vi "BCU参数读取-Auto.vi"(8 "CAN端口":u16(ring), 9 "设备索引号":u16(ring), 10 "CAN卡类型":u32(ring)=21, 11 "Myindex":dbl=1.0) -> (3 "成功":bool)   [LabVIEW 2013] (continued)
                        n3743 = Boolean To (0,1)(Boolean=w5434) -> (0, 1=w5432:i16)
                        n3744 = Quotient & Remainder(x=w5429, y=w5430) -> (x-y*floor(x/y)=w5426:dbl)  [unwired: 1 out]
                        n3745 = Build Array(i16 170 ("元素"), w5432, w5426, w5425, w5424, w5423, 0.0 ("元素")) -> (w5435:dbl[])
                        n3746 = call "多帧发送机制(EV05).vi"("can卡类型"=w5439, "设备索引号"=w5438, "CAN端口"=w5437, "命令"=w5420, "板号"=u8 0, "命令序号"=w5421, "输入数据"=w5435) -> ()  [unwired: 2 in, 11 out]
                        n3747 = local write "命令序号"(w5421) -> ()
                        n3748 = local write "命令"(w5420) -> ()
                      }
                    }
                    n3749 = local write "控制1"(TRUE ("控制1")) -> ()
                    n3750 = local write "写?"(FALSE ("写?")) -> ()
                    n3751 = local write "消除"(TRUE ("消除")) -> ()
                    n3752 = global write "EV05全局变量1.vi" "流控帧 2"(TRUE ("流控帧 2")) -> ()
                    n3753 = global write "EV05全局变量1.vi" "流控帧"(FALSE ("流控帧")) -> ()
                  }
                  frame #2 {
                    n3754 = flat-sequence {
                      tunnel: [w5441] -> w5440
                      tunnel: w5440 -> [w5448]
                      frame #0 {
                        n3755 = while {
                          tunnel: [w5442] -> w5441
                          i -> [w5446]
                          stop <- w5443 stop-if-true
                          n3756 = local read "继电器超时处理"() -> (w5442:bool)
                          n3757 = Greater Or Equal?(x=w5446, y=20) -> (x >= y?=w5444:bool)
                          n3758 = Wait Until Next ms Multiple(millisecond multiple=u32 100 ("毫秒倍数")) -> ()  [unwired: 1 out]
                          n3759 = Or(x=w5442, y=w5444) -> (x .or. y?=w5443:bool)
                        }
                      }
                      frame #1 {
                        n3760 = case shown="真" w5448 {
                          frame False {
                            n3761 = One Button Dialog(message="继电器处理超时" ("消息"), button name ("OK")="是" ("按钮名称（“确定”）")) -> ()  [unwired: 1 out]
                          }
                          frame True {
                            w5451 = TRUE ("清BUFF")
                            n3762 = local write "正级继电器"(w5451) -> ()
                            n3763 = local write "负级继电器"(w5451) -> ()
                            n3764 = local write "充电继电器"(w5451) -> ()
                            n3765 = local write "加热继电器"(w5451) -> ()
                            n3766 = local write "风机继电器"(w5451) -> ()
                            n3767 = local write "预充电继电器"(w5451) -> ()
                          }
                        }
                      }
                    }
                  }
                }
              }
            }
          }
          event "继电器全关": Value Change {
            n3768 = event-data() -> ("NewVal"=w5452:bool)  [unwired: 6 out]
            n3769 = case shown="真" w5452 {
              tunnel: w5452 -> [_ w5455]
              frame False {
              }
              frame True {
                n3770 = stacked-sequence {
                  tunnel: w5455 -> [_ w5465 _]
                  frame #0 {
                    w5456 = TRUE ("清BUFF")
                    n3771 = local write "正级继电器"(w5456) -> ()
                    n3772 = local write "负级继电器"(w5456) -> ()
                    n3773 = local write "充电继电器"(w5456) -> ()
                    n3774 = local write "加热继电器"(w5456) -> ()
                    n3775 = local write "风机继电器"(w5456) -> ()
                    n3776 = local write "预充电继电器"(w5456) -> ()
                    n3777 = local write "继电器超时处理"(FALSE ("继电器超时处理")) -> ()
                    n3778 = local write "主从选择"(enum32{"主板", "从板"}."主板" ("主从选择")) -> ()
                    n3779 = global write "EV05全局变量1.vi" "流控帧"(FALSE ("流控帧")) -> ()
                    n3780 = local write "清BUFF"(FALSE ("清BUFF")) -> ()
                  }
                  frame #1 {
                    n3781 = case shown="真" w5465 {
                      selector: w5465 -> [_ w5480]
                      frame False {
                      }
                      frame True {
                        w5476 = 256.0 ("y")
                        w5467 = u32 1 ("命令序号")
                        w5466 = u8 192 ("命令")
                        n3782 = local read "动作保持时间"() -> (w5477:dbl)
                        n3783 = Quotient & Remainder(x=w5477, y=w5476) -> (x-y*floor(x/y)=w5469:dbl, floor(x/y)=w5473:dbl)
                        n3784 = Quotient & Remainder(x=w5473, y=w5476) -> (x-y*floor(x/y)=w5470:dbl, floor(x/y)=w5474:dbl)
                        n3785 = Quotient & Remainder(x=w5474, y=w5476) -> (x-y*floor(x/y)=w5471:dbl, floor(x/y)=w5475:dbl)
                        n3786 = local read "设备索引号"() -> (w5484:u16)
                        n3787 = local read "CAN卡类型"() -> (w5485:u32)
                        n3788 = local read "CAN端口"() -> (w5483:u16)
                        n3789 = Boolean To (0,1)(Boolean=w5480) -> (0, 1=w5478:i16)
                        n3790 = Quotient & Remainder(x=w5475, y=w5476) -> (x-y*floor(x/y)=w5472:dbl)  [unwired: 1 out]
                        n3791 = Build Array(i16 85 ("元素"), w5478, w5472, w5471, w5470, w5469, 0.0 ("元素")) -> (w5481:dbl[])
                        n3792 = call "多帧发送机制(EV05).vi"("can卡类型"=w5485, "设备索引号"=w5484, "CAN端口"=w5483, "命令"=w5466, "板号"=u8 0, "命令序号"=w5467, "输入数据"=w5481) -> ()  [unwired: 2 in, 11 out]
                        n3793 = local write "命令序号"(w5467) -> ()
                        n3794 = local write "命令"(w5466) -> ()
                      }
                    }
                    n3795 = local write "控制1"(TRUE ("控制1")) -> ()
                    n3796 = local write "写?"(FALSE ("写?")) -> ()
                    n3797 = local write "消除"(TRUE ("消除")) -> ()
                    n3798 = global write "EV05全局变量1.vi" "流控帧 2"(TRUE ("流控帧 2")) -> ()
                  }
                  frame #2 {
                    n3799 = flat-sequence {
                      tunnel: [w5487] -> w5486
                      tunnel: w5486 -> [w5494]
                      frame #0 {
                        n3800 = while {
                          tunnel: [w5488] -> w5487
                          i -> [w5492]
                          stop <- w5489 stop-if-true
                          n3801 = local read "继电器超时处理"() -> (w5488:bool)
                          n3802 = Greater Or Equal?(x=w5492, y=20) -> (x >= y?=w5490:bool)
                          n3803 = Wait Until Next ms Multiple(millisecond multiple=u32 100 ("毫秒倍数")) -> ()  [unwired: 1 out]
                          n3804 = Or(x=w5488, y=w5490) -> (x .or. y?=w5489:bool)
                        }
                      }
                      frame #1 {
                        n3805 = case shown="真" w5494 {
                          frame False {
                            n3806 = One Button Dialog(message="继电器处理超时" ("消息"), button name ("OK")="是" ("按钮名称（“确定”）")) -> ()  [unwired: 1 out]
                          }
                          frame True {
                            w5497 = FALSE ("清BUFF")
                            n3807 = local write "正级继电器"(w5497) -> ()
                            n3808 = local write "负级继电器"(w5497) -> ()
                            n3809 = local write "充电继电器"(w5497) -> ()
                            n3810 = local write "加热继电器"(w5497) -> ()
                            n3811 = local write "风机继电器"(w5497) -> ()
                            n3812 = local write "预充电继电器"(w5497) -> ()
                          }
                        }
                      }
                    }
                  }
                }
              }
            }
          }
          event "控制按键全为开": Value Change {
            n3813 = event-data() -> ("NewVal"=w5498:bool)  [unwired: 6 out]
            n3814 = case shown="真" w5498 {
              frame False {
              }
              frame True {
                w5499 = TRUE ("正级继电器")
                n3815 = local write "加热继电器(从)"(w5499) -> ()
                n3816 = local write "风机继电器(从)"(w5499) -> ()
                n3817 = local write "DO1 2"(w5499) -> ()
                n3818 = local write "DO1"(w5499) -> ()
                n3819 = local write "DO2"(w5499) -> ()
                n3820 = local write "正级继电器"(w5499) -> ()
                n3821 = local write "负级继电器"(w5499) -> ()
                n3822 = local write "加热继电器"(w5499) -> ()
                n3823 = local write "预充电继电器"(w5499) -> ()
                n3824 = local write "充电继电器"(w5499) -> ()
                n3825 = local write "风机继电器"(w5499) -> ()
              }
            }
          }
          event "控制按键全为关": Value Change {
            n3826 = event-data() -> ("NewVal"=w5500:bool)  [unwired: 6 out]
            n3827 = case shown="真" w5500 {
              frame False {
              }
              frame True {
                w5501 = FALSE ("正级继电器")
                n3828 = local write "加热继电器(从)"(w5501) -> ()
                n3829 = local write "风机继电器(从)"(w5501) -> ()
                n3830 = local write "DO1 2"(w5501) -> ()
                n3831 = local write "DO1"(w5501) -> ()
                n3832 = local write "DO2"(w5501) -> ()
                n3833 = local write "正级继电器"(w5501) -> ()
                n3834 = local write "负级继电器"(w5501) -> ()
                n3835 = local write "加热继电器"(w5501) -> ()
                n3836 = local write "预充电继电器"(w5501) -> ()
                n3837 = local write "充电继电器"(w5501) -> ()
                n3838 = local write "风机继电器"(w5501) -> ()
              }
            }
          }
          event "正级继电器": Value Change {
            n3839 = event-data() -> ("NewVal"=w5502:bool)  [unwired: 6 out]
            n3840 = stacked-sequence {
              tunnel: w5502 -> [_ w5515 _]
              frame #0 {
                w5505 = FALSE ("清BUFF")
                n3841 = local write "继电器超时处理"(FALSE ("继电器超时处理")) -> ()
                n3842 = local write "主从选择"(enum32{"主板", "从板"}."主板" ("主从选择")) -> ()
                n3843 = local write "正级继电器 12"(w5505) -> ()
                n3844 = local write "清BUFF"(w5505) -> ()
              }
              frame #1 {
                n3845 = case shown="假" w5515 {
                  selector: w5515 -> [w5530 w5550]
                  tunnel: [w5529 w5549] -> w5514
                  tunnel: [w5517 w5537] -> w5509
                  frame False {
                    w5525 = 256.0 ("y")
                    w5517 = u32 1 ("命令序号")
                    w5529 = u8 192 ("命令")
                    n3846 = local read "动作保持时间"() -> (w5526:dbl)
                    n3847 = Quotient & Remainder(x=w5526, y=w5525) -> (x-y*floor(x/y)=w5518:dbl, floor(x/y)=w5522:dbl)
                    n3848 = Quotient & Remainder(x=w5522, y=w5525) -> (x-y*floor(x/y)=w5519:dbl, floor(x/y)=w5523:dbl)
                    n3849 = Quotient & Remainder(x=w5523, y=w5525) -> (x-y*floor(x/y)=w5520:dbl, floor(x/y)=w5524:dbl)
                    n3850 = local read "设备索引号"() -> (w5534:u16)
                    n3851 = local read "CAN卡类型"() -> (w5535:u32)
                    n3852 = local read "CAN端口"() -> (w5533:u16)
                    n3853 = Boolean To (0,1)(Boolean=w5530) -> (0, 1=w5527:i16)
                    n3854 = Quotient & Remainder(x=w5524, y=w5525) -> (x-y*floor(x/y)=w5521:dbl)  [unwired: 1 out]
                    n3855 = Build Array(i16 1 ("元素"), w5527, w5521, w5520, w5519, w5518, 0.0 ("元素")) -> (w5531:dbl[])
                    n3856 = call "多帧发送机制(EV05).vi"("can卡类型"=w5535, "设备索引号"=w5534, "CAN端口"=w5533, "命令"=w5529, "板号"=u8 0, "命令序号"=w5517, "输入数据"=w5531) -> ()  [unwired: 2 in, 11 out]
                  }
                  frame True {
                    w5545 = 256.0 ("y")
                    w5537 = u32 1 ("命令序号")
                    w5549 = u8 192 ("命令")
                    n3857 = local read "动作保持时间"() -> (w5546:dbl)
                    n3858 = Quotient & Remainder(x=w5546, y=w5545) -> (x-y*floor(x/y)=w5538:dbl, floor(x/y)=w5542:dbl)
                    n3859 = Quotient & Remainder(x=w5542, y=w5545) -> (x-y*floor(x/y)=w5539:dbl, floor(x/y)=w5543:dbl)
                    n3860 = Quotient & Remainder(x=w5543, y=w5545) -> (x-y*floor(x/y)=w5540:dbl, floor(x/y)=w5544:dbl)
                    n3861 = local read "设备索引号"() -> (w5554:u16)
                    n3862 = local read "CAN卡类型"() -> (w5555:u32)
                    n3863 = local read "CAN端口"() -> (w5553:u16)
                    n3864 = Boolean To (0,1)(Boolean=w5550) -> (0, 1=w5547:i16)
                    n3865 = Quotient & Remainder(x=w5544, y=w5545) -> (x-y*floor(x/y)=w5541:dbl)  [unwired: 1 out]
                    n3866 = Build Array(i16 1 ("元素"), w5547, w5541, w5540, w5539, w5538, 0.0 ("元素")) -> (w5551:dbl[])
                    n3867 = call "多帧发送机制(EV05).vi"("can卡类型"=w5555, "设备索引号"=w5554, "CAN端口"=w5553, "命令"=w5549, "板号"=u8 0, "命令序号"=w5537, "输入数据"=w5551) -> ()  [unwired: 2 in, 11 out]
                  }
                }
                n3868 = local write "命令序号"(w5509) -> ()
                n3869 = local write "命令"(w5514) -> ()
                n3870 = local write "控制1"(TRUE ("控制1")) -> ()
                n3871 = local write "写?"(FALSE ("写?")) -> ()
                n3872 = global write "EV05全局变量1.vi" "流控帧"(FALSE ("流控帧")) -> ()
                n3873 = local write "消除"(TRUE ("消除")) -> ()
                n3874 = global write "EV05全局变量1.vi" "流控帧 2"(TRUE ("流控帧 2")) -> ()
              }
              frame #2 {
                n3875 = flat-sequence {
                  tunnel: [w5557] -> w5556
                  tunnel: w5556 -> [w5564]
                  frame #0 {
                    n3876 = while {
                      tunnel: [w5558] -> w5557
                      i -> [w5562]
                      stop <- w5559 stop-if-true
                      n3877 = local read "继电器超时处理"() -> (w5558:bool)
                      n3878 = Greater Or Equal?(x=w5562, y=20) -> (x >= y?=w5560:bool)
                      n3879 = Wait Until Next ms Multiple(millisecond multiple=u32 100 ("毫秒倍数")) -> ()  [unwired: 1 out]
                      n3880 = Or(x=w5558, y=w5560) -> (x .or. y?=w5559:bool)
                    }
                  }
                  frame #1 {
                    n3881 = case shown="假" w5564 {
                      frame False {
                        n3882 = local read "正级继电器"() -> (w5566:bool)
                        n3883 = Not(x=w5566) -> (.not. x?=w5565:bool)
                        n3884 = local write "正级继电器"(w5565) -> ()
                        n3885 = One Button Dialog(message="继电器处理超时" ("消息"), button name ("OK")="是" ("按钮名称（“确定”）")) -> ()  [unwired: 1 out]
                      }
                      frame True {
                      }
                    }
                  }
                }
              }
            }
          }
          event "负级继电器": Value Change {
            n3886 = event-data() -> ("NewVal"=w5569:bool)  [unwired: 6 out]
            n3887 = stacked-sequence {
              tunnel: w5569 -> [_ w5582 _]
              frame #0 {
                w5572 = FALSE ("继电器超时处理")
                n3888 = local write "继电器超时处理"(w5572) -> ()
                n3889 = local write "正级继电器 2"(w5572) -> ()
                n3890 = local write "主从选择"(enum32{"主板", "从板"}."主板" ("主从选择")) -> ()
              }
              frame #1 {
                n3891 = case shown="假" w5582 {
                  selector: w5582 -> [w5596 w5616]
                  tunnel: [w5595 w5615] -> w5581
                  tunnel: [w5584 w5604] -> w5576
                  frame False {
                    w5592 = 256.0 ("y")
                    w5584 = u32 1 ("命令序号")
                    w5595 = u8 192 ("命令")
                    n3892 = local read "动作保持时间"() -> (w5593:dbl)
                    n3893 = Quotient & Remainder(x=w5593, y=w5592) -> (x-y*floor(x/y)=w5585:dbl, floor(x/y)=w5589:dbl)
                    n3894 = Quotient & Remainder(x=w5589, y=w5592) -> (x-y*floor(x/y)=w5586:dbl, floor(x/y)=w5590:dbl)
                    n3895 = Quotient & Remainder(x=w5590, y=w5592) -> (x-y*floor(x/y)=w5587:dbl, floor(x/y)=w5591:dbl)
                    n3896 = Quotient & Remainder(x=w5591, y=w5592) -> (x-y*floor(x/y)=w5588:dbl)  [unwired: 1 out]
                    n3897 = Boolean To (0,1)(Boolean=w5596) -> (0, 1=w5594:i16)
                    n3898 = local read "设备索引号"() -> (w5601:u16)
                    n3899 = local read "CAN卡类型"() -> (w5602:u32)
                    n3900 = local read "CAN端口"() -> (w5600:u16)
                    n3901 = Build Array(i16 2 ("元素"), w5594, w5588, w5587, w5586, w5585, 0.0 ("元素")) -> (w5598:dbl[])
                    n3902 = call "多帧发送机制(EV05).vi"("can卡类型"=w5602, "设备索引号"=w5601, "CAN端口"=w5600, "命令"=w5595, "板号"=u8 0, "命令序号"=w5584, "输入数据"=w5598) -> ()  [unwired: 2 in, 11 out]
                  }
                  frame True {
                    w5612 = 256.0 ("y")
                    w5604 = u32 1 ("命令序号")
                    w5615 = u8 192 ("命令")
                    n3903 = local read "动作保持时间"() -> (w5613:dbl)
                    n3904 = Quotient & Remainder(x=w5613, y=w5612) -> (x-y*floor(x/y)=w5605:dbl, floor(x/y)=w5609:dbl)
                    n3905 = Quotient & Remainder(x=w5609, y=w5612) -> (x-y*floor(x/y)=w5606:dbl, floor(x/y)=w5610:dbl)
                    n3906 = Quotient & Remainder(x=w5610, y=w5612) -> (x-y*floor(x/y)=w5607:dbl, floor(x/y)=w5611:dbl)
                    n3907 = Quotient & Remainder(x=w5611, y=w5612) -> (x-y*floor(x/y)=w5608:dbl)  [unwired: 1 out]
                    n3908 = Boolean To (0,1)(Boolean=w5616) -> (0, 1=w5614:i16)
                    n3909 = local read "设备索引号"() -> (w5621:u16)
                    n3910 = local read "CAN卡类型"() -> (w5622:u32)
                    n3911 = local read "CAN端口"() -> (w5620:u16)
                    n3912 = Build Array(i16 2 ("元素"), w5614, w5608, w5607, w5606, w5605, 0.0 ("元素")) -> (w5618:dbl[])
                    n3913 = call "多帧发送机制(EV05).vi"("can卡类型"=w5622, "设备索引号"=w5621, "CAN端口"=w5620, "命令"=w5615, "板号"=u8 0, "命令序号"=w5604, "输入数据"=w5618) -> ()  [unwired: 2 in, 11 out]
                  }
                }
                n3914 = local write "命令"(w5581) -> ()
                n3915 = local write "命令序号"(w5576) -> ()
                n3916 = local write "清BUFF"(FALSE ("清BUFF")) -> ()
                n3917 = global write "EV05全局变量1.vi" "流控帧"(FALSE ("流控帧")) -> ()
                n3918 = local write "控制1"(TRUE ("控制1")) -> ()
                n3919 = global write "EV05全局变量1.vi" "流控帧 2"(TRUE ("流控帧 2")) -> ()
                n3920 = local write "写?"(FALSE ("写?")) -> ()
                n3921 = local write "消除"(TRUE ("消除")) -> ()
              }
              frame #2 {
                n3922 = flat-sequence {
                  tunnel: [w5624] -> w5623
                  tunnel: w5623 -> [w5631]
                  frame #0 {
                    n3923 = while {
                      tunnel: [w5625] -> w5624
                      i -> [w5629]
                      stop <- w5626 stop-if-true
                      n3924 = local read "继电器超时处理"() -> (w5625:bool)
                      n3925 = Greater Or Equal?(x=w5629, y=20) -> (x >= y?=w5627:bool)
                      n3926 = Wait Until Next ms Multiple(millisecond multiple=u32 100 ("毫秒倍数")) -> ()  [unwired: 1 out]
                      n3927 = Or(x=w5625, y=w5627) -> (x .or. y?=w5626:bool)
                    }
                  }
                  frame #1 {
                    n3928 = case shown="假" w5631 {
                      frame False {
                        n3929 = local read "负级继电器"() -> (w5632:bool)
                        n3930 = Not(x=w5632) -> (.not. x?=w5633:bool)
                        n3931 = local write "负级继电器"(w5633) -> ()
                        n3932 = One Button Dialog(message="继电器处理超时" ("消息"), button name ("OK")="是" ("按钮名称（“确定”）")) -> ()  [unwired: 1 out]
                      }
                      frame True {
                      }
                    }
                  }
                }
              }
            }
          }
          event "预充电继电器": Value Change {
            n3933 = event-data() -> ("NewVal"=w5636:bool)  [unwired: 6 out]
            n3934 = stacked-sequence {
              tunnel: w5636 -> [_ w5649 _]
              frame #0 {
                w5640 = FALSE ("继电器超时处理")
                n3935 = local write "继电器超时处理"(w5640) -> ()
                n3936 = local write "正级继电器 3"(w5640) -> ()
                n3937 = global write "EV05全局变量1.vi" "流控帧"(FALSE ("流控帧")) -> ()
                n3938 = local write "主从选择"(enum32{"主板", "从板"}."主板" ("主从选择")) -> ()
              }
              frame #1 {
                n3939 = case shown="假" w5649 {
                  selector: w5649 -> [w5663 w5683]
                  tunnel: [w5662 w5682] -> w5648
                  tunnel: [w5651 w5671] -> w5643
                  frame False {
                    w5659 = 256.0 ("y")
                    w5651 = u32 1 ("命令序号")
                    w5662 = u8 192 ("命令")
                    n3940 = local read "动作保持时间"() -> (w5660:dbl)
                    n3941 = Quotient & Remainder(x=w5660, y=w5659) -> (x-y*floor(x/y)=w5652:dbl, floor(x/y)=w5656:dbl)
                    n3942 = Quotient & Remainder(x=w5656, y=w5659) -> (x-y*floor(x/y)=w5653:dbl, floor(x/y)=w5657:dbl)
                    n3943 = Quotient & Remainder(x=w5657, y=w5659) -> (x-y*floor(x/y)=w5654:dbl, floor(x/y)=w5658:dbl)
                    n3944 = Quotient & Remainder(x=w5658, y=w5659) -> (x-y*floor(x/y)=w5655:dbl)  [unwired: 1 out]
                    n3945 = Boolean To (0,1)(Boolean=w5663) -> (0, 1=w5661:i16)
                    n3946 = local read "设备索引号"() -> (w5668:u16)
                    n3947 = local read "CAN卡类型"() -> (w5669:u32)
                    n3948 = local read "CAN端口"() -> (w5667:u16)
                    n3949 = Build Array(i16 3 ("元素"), w5661, w5655, w5654, w5653, w5652, 0.0 ("元素")) -> (w5665:dbl[])
                    n3950 = call "多帧发送机制(EV05).vi"("can卡类型"=w5669, "设备索引号"=w5668, "CAN端口"=w5667, "命令"=w5662, "板号"=u8 0, "命令序号"=w5651, "输入数据"=w5665) -> ()  [unwired: 2 in, 11 out]
                  }
                  frame True {
                    w5679 = 256.0 ("y")
                    w5671 = u32 1 ("命令序号")
                    w5682 = u8 192 ("命令")
                    n3951 = local read "动作保持时间"() -> (w5680:dbl)
                    n3952 = Quotient & Remainder(x=w5680, y=w5679) -> (x-y*floor(x/y)=w5672:dbl, floor(x/y)=w5676:dbl)
                    n3953 = Quotient & Remainder(x=w5676, y=w5679) -> (x-y*floor(x/y)=w5673:dbl, floor(x/y)=w5677:dbl)
                    n3954 = Quotient & Remainder(x=w5677, y=w5679) -> (x-y*floor(x/y)=w5674:dbl, floor(x/y)=w5678:dbl)
                    n3955 = Quotient & Remainder(x=w5678, y=w5679) -> (x-y*floor(x/y)=w5675:dbl)  [unwired: 1 out]
                    n3956 = Boolean To (0,1)(Boolean=w5683) -> (0, 1=w5681:i16)
                    n3957 = local read "设备索引号"() -> (w5688:u16)
                    n3958 = local read "CAN卡类型"() -> (w5689:u32)
                    n3959 = local read "CAN端口"() -> (w5687:u16)
                    n3960 = Build Array(i16 3 ("元素"), w5681, w5675, w5674, w5673, w5672, 0.0 ("元素")) -> (w5685:dbl[])
                    n3961 = call "多帧发送机制(EV05).vi"("can卡类型"=w5689, "设备索引号"=w5688, "CAN端口"=w5687, "命令"=w5682, "板号"=u8 0, "命令序号"=w5671, "输入数据"=w5685) -> ()  [unwired: 2 in, 11 out]
                  }
                }
                n3962 = local write "命令序号"(w5643) -> ()
                n3963 = local write "清BUFF"(FALSE ("清BUFF")) -> ()
                n3964 = local write "控制1"(TRUE ("控制1")) -> ()
                n3965 = global write "EV05全局变量1.vi" "流控帧 2"(TRUE ("流控帧 2")) -> ()
                n3966 = local write "消除"(TRUE ("消除")) -> ()
                n3967 = local write "命令"(w5648) -> ()
                n3968 = local write "写?"(FALSE ("写?")) -> ()
              }
              frame #2 {
                n3969 = flat-sequence {
                  tunnel: [w5691] -> w5690
                  tunnel: w5690 -> [w5698]
                  frame #0 {
                    n3970 = while {
                      tunnel: [w5692] -> w5691
                      i -> [w5696]
                      stop <- w5693 stop-if-true
                      n3971 = local read "继电器超时处理"() -> (w5692:bool)
                      n3972 = Greater Or Equal?(x=w5696, y=20) -> (x >= y?=w5694:bool)
                      n3973 = Wait Until Next ms Multiple(millisecond multiple=u32 100 ("毫秒倍数")) -> ()  [unwired: 1 out]
                      n3974 = Or(x=w5692, y=w5694) -> (x .or. y?=w5693:bool)
                    }
                  }
                  frame #1 {
                    n3975 = case shown="假" w5698 {
                      frame False {
                        n3976 = local read "预充电继电器"() -> (w5699:bool)
                        n3977 = Not(x=w5699) -> (.not. x?=w5700:bool)
                        n3978 = local write "预充电继电器"(w5700) -> ()
                        n3979 = One Button Dialog(message="继电器处理超时" ("消息"), button name ("OK")="是" ("按钮名称（“确定”）")) -> ()  [unwired: 1 out]
                      }
                      frame True {
                      }
                    }
                  }
                }
              }
            }
          }
          event "加热继电器": Value Change {
            n3980 = event-data() -> ("NewVal"=w5703:bool)  [unwired: 6 out]
            n3981 = stacked-sequence {
              tunnel: w5703 -> [_ w5716 _]
              frame #0 {
                w5707 = FALSE ("继电器超时处理")
                n3982 = local write "继电器超时处理"(w5707) -> ()
                n3983 = local write "正级继电器 5"(w5707) -> ()
                n3984 = global write "EV05全局变量1.vi" "流控帧"(FALSE ("流控帧")) -> ()
                n3985 = local write "主从选择"(enum32{"主板", "从板"}."主板" ("主从选择")) -> ()
              }
              frame #1 {
                n3986 = case shown="假" w5716 {
                  selector: w5716 -> [w5730 w5750]
                  tunnel: [w5729 w5749] -> w5715
                  tunnel: [w5718 w5738] -> w5710
                  frame False {
                    w5726 = 256.0 ("y")
                    w5718 = u32 1 ("命令序号")
                    w5729 = u8 192 ("命令")
                    n3987 = local read "动作保持时间"() -> (w5727:dbl)
                    n3988 = Quotient & Remainder(x=w5727, y=w5726) -> (x-y*floor(x/y)=w5719:dbl, floor(x/y)=w5723:dbl)
                    n3989 = Quotient & Remainder(x=w5723, y=w5726) -> (x-y*floor(x/y)=w5720:dbl, floor(x/y)=w5724:dbl)
                    n3990 = Quotient & Remainder(x=w5724, y=w5726) -> (x-y*floor(x/y)=w5721:dbl, floor(x/y)=w5725:dbl)
                    n3991 = Quotient & Remainder(x=w5725, y=w5726) -> (x-y*floor(x/y)=w5722:dbl)  [unwired: 1 out]
                    n3992 = Boolean To (0,1)(Boolean=w5730) -> (0, 1=w5728:i16)
                    n3993 = local read "设备索引号"() -> (w5735:u16)
                    n3994 = local read "CAN卡类型"() -> (w5736:u32)
                    n3995 = local read "CAN端口"() -> (w5734:u16)
                    n3996 = Build Array(i16 4 ("元素"), w5728, w5722, w5721, w5720, w5719, 0.0 ("元素")) -> (w5732:dbl[])
                    n3997 = call "多帧发送机制(EV05).vi"("can卡类型"=w5736, "设备索引号"=w5735, "CAN端口"=w5734, "命令"=w5729, "板号"=u8 0, "命令序号"=w5718, "输入数据"=w5732) -> ()  [unwired: 2 in, 11 out]
                  }
                  frame True {
                    w5746 = 256.0 ("y")
                    w5738 = u32 1 ("命令序号")
                    w5749 = u8 192 ("命令")
                    n3998 = local read "动作保持时间"() -> (w5747:dbl)
                    n3999 = Quotient & Remainder(x=w5747, y=w5746) -> (x-y*floor(x/y)=w5739:dbl, floor(x/y)=w5743:dbl)
                    n4000 = Quotient & Remainder(x=w5743, y=w5746) -> (x-y*floor(x/y)=w5740:dbl, floor(x/y)=w5744:dbl)
                    n4001 = Quotient & Remainder(x=w5744, y=w5746) -> (x-y*floor(x/y)=w5741:dbl, floor(x/y)=w5745:dbl)
                    n4002 = Quotient & Remainder(x=w5745, y=w5746) -> (x-y*floor(x/y)=w5742:dbl)  [unwired: 1 out]
                    n4003 = Boolean To (0,1)(Boolean=w5750) -> (0, 1=w5748:i16)
                    n4004 = local read "设备索引号"() -> (w5755:u16)
                    n4005 = local read "CAN卡类型"() -> (w5756:u32)
                    n4006 = local read "CAN端口"() -> (w5754:u16)
                    n4007 = Build Array(i16 4 ("元素"), w5748, w5742, w5741, w5740, w5739, 0.0 ("元素")) -> (w5752:dbl[])
                    n4008 = call "多帧发送机制(EV05).vi"("can卡类型"=w5756, "设备索引号"=w5755, "CAN端口"=w5754, "命令"=w5749, "板号"=u8 0, "命令序号"=w5738, "输入数据"=w5752) -> ()  [unwired: 2 in, 11 out]
                  }
                }
                n4009 = local write "命令序号"(w5710) -> ()
                n4010 = local write "清BUFF"(FALSE ("清BUFF")) -> ()
                n4011 = local write "命令"(w5715) -> ()
                n4012 = local write "控制1"(TRUE ("控制1")) -> ()
                n4013 = local write "写?"(FALSE ("写?")) -> ()
                n4014 = global write "EV05全局变量1.vi" "流控帧 2"(TRUE ("流控帧 2")) -> ()
                n4015 = local write "消除"(TRUE ("消除")) -> ()
              }
              frame #2 {
                n4016 = flat-sequence {
                  tunnel: [w5758] -> w5757
                  tunnel: w5757 -> [w5765]
                  frame #0 {
                    n4017 = while {
                      tunnel: [w5759] -> w5758
                      i -> [w5763]
                      stop <- w5760 stop-if-true
                      n4018 = local read "继电器超时处理"() -> (w5759:bool)
                      n4019 = Greater Or Equal?(x=w5763, y=20) -> (x >= y?=w5761:bool)
                      n4020 = Wait Until Next ms Multiple(millisecond multiple=u32 100 ("毫秒倍数")) -> ()  [unwired: 1 out]
                      n4021 = Or(x=w5759, y=w5761) -> (x .or. y?=w5760:bool)
                    }
                  }
                  frame #1 {
                    n4022 = case shown="假" w5765 {
                      frame False {
                        n4023 = local read "加热继电器"() -> (w5766:bool)
                        n4024 = Not(x=w5766) -> (.not. x?=w5767:bool)
                        n4025 = local write "加热继电器"(w5767) -> ()
                        n4026 = One Button Dialog(message="继电器处理超时" ("消息"), button name ("OK")="是" ("按钮名称（“确定”）")) -> ()  [unwired: 1 out]
                      }
                      frame True {
                      }
                    }
                  }
                }
              }
            }
          }
          event "充电继电器": Value Change {
            n4027 = event-data() -> ("NewVal"=w5770:bool)  [unwired: 6 out]
            n4028 = stacked-sequence {
              tunnel: w5770 -> [_ w5783 _]
              frame #0 {
                w5774 = FALSE ("继电器超时处理")
                n4029 = local write "主从选择"(enum32{"主板", "从板"}."主板" ("主从选择")) -> ()
                n4030 = global write "EV05全局变量1.vi" "流控帧"(FALSE ("流控帧")) -> ()
                n4031 = local write "继电器超时处理"(w5774) -> ()
                n4032 = local write "正级继电器 4"(w5774) -> ()
              }
              frame #1 {
                n4033 = case shown="假" w5783 {
                  selector: w5783 -> [w5797 w5817]
                  tunnel: [w5796 w5816] -> w5782
                  tunnel: [w5785 w5805] -> w5777
                  frame False {
                    w5793 = 256.0 ("y")
                    w5785 = u32 1 ("命令序号")
                    w5796 = u8 192 ("命令")
                    n4034 = local read "动作保持时间"() -> (w5794:dbl)
                    n4035 = Quotient & Remainder(x=w5794, y=w5793) -> (x-y*floor(x/y)=w5786:dbl, floor(x/y)=w5790:dbl)
                    n4036 = Quotient & Remainder(x=w5790, y=w5793) -> (x-y*floor(x/y)=w5787:dbl, floor(x/y)=w5791:dbl)
                    n4037 = Quotient & Remainder(x=w5791, y=w5793) -> (x-y*floor(x/y)=w5788:dbl, floor(x/y)=w5792:dbl)
                    n4038 = Quotient & Remainder(x=w5792, y=w5793) -> (x-y*floor(x/y)=w5789:dbl)  [unwired: 1 out]
                    n4039 = Boolean To (0,1)(Boolean=w5797) -> (0, 1=w5795:i16)
                    n4040 = local read "设备索引号"() -> (w5802:u16)
                    n4041 = local read "CAN卡类型"() -> (w5803:u32)
                    n4042 = local read "CAN端口"() -> (w5801:u16)
                    n4043 = Build Array(i16 5 ("元素"), w5795, w5789, w5788, w5787, w5786, 0.0 ("元素")) -> (w5799:dbl[])
                    n4044 = call "多帧发送机制(EV05).vi"("can卡类型"=w5803, "设备索引号"=w5802, "CAN端口"=w5801, "命令"=w5796, "板号"=u8 0, "命令序号"=w5785, "输入数据"=w5799) -> ()  [unwired: 2 in, 11 out]
                  }
                  frame True {
                    w5813 = 256.0 ("y")
                    w5805 = u32 1 ("命令序号")
                    w5816 = u8 192 ("命令")
                    n4045 = local read "动作保持时间"() -> (w5814:dbl)
                    n4046 = Quotient & Remainder(x=w5814, y=w5813) -> (x-y*floor(x/y)=w5806:dbl, floor(x/y)=w5810:dbl)
                    n4047 = Quotient & Remainder(x=w5810, y=w5813) -> (x-y*floor(x/y)=w5807:dbl, floor(x/y)=w5811:dbl)
                    n4048 = Quotient & Remainder(x=w5811, y=w5813) -> (x-y*floor(x/y)=w5808:dbl, floor(x/y)=w5812:dbl)
                    n4049 = Quotient & Remainder(x=w5812, y=w5813) -> (x-y*floor(x/y)=w5809:dbl)  [unwired: 1 out]
                    n4050 = Boolean To (0,1)(Boolean=w5817) -> (0, 1=w5815:i16)
                    n4051 = local read "设备索引号"() -> (w5822:u16)
                    n4052 = local read "CAN卡类型"() -> (w5823:u32)
                    n4053 = local read "CAN端口"() -> (w5821:u16)
                    n4054 = Build Array(i16 5 ("元素"), w5815, w5809, w5808, w5807, w5806, 0.0 ("元素")) -> (w5819:dbl[])
                    n4055 = call "多帧发送机制(EV05).vi"("can卡类型"=w5823, "设备索引号"=w5822, "CAN端口"=w5821, "命令"=w5816, "板号"=u8 0, "命令序号"=w5805, "输入数据"=w5819) -> ()  [unwired: 2 in, 11 out]
                  }
                }
                n4056 = local write "命令序号"(w5777) -> ()
                n4057 = local write "命令"(w5782) -> ()
                n4058 = local write "清BUFF"(FALSE ("清BUFF")) -> ()
                n4059 = local write "控制1"(TRUE ("控制1")) -> ()
                n4060 = global write "EV05全局变量1.vi" "流控帧 2"(TRUE ("流控帧 2")) -> ()
                n4061 = local write "写?"(FALSE ("写?")) -> ()
                n4062 = local write "消除"(TRUE ("消除")) -> ()
              }
              frame #2 {
                n4063 = flat-sequence {
                  tunnel: [w5825] -> w5824
                  tunnel: w5824 -> [w5832]
                  frame #0 {
                    n4064 = while {
                      tunnel: [w5826] -> w5825
                      i -> [w5830]
                      stop <- w5827 stop-if-true
                      n4065 = local read "继电器超时处理"() -> (w5826:bool)
                      n4066 = Greater Or Equal?(x=w5830, y=20) -> (x >= y?=w5828:bool)
                      n4067 = Wait Until Next ms Multiple(millisecond multiple=u32 100 ("毫秒倍数")) -> ()  [unwired: 1 out]
                      n4068 = Or(x=w5826, y=w5828) -> (x .or. y?=w5827:bool)
                    }
                  }
                  frame #1 {
                    n4069 = case shown="假" w5832 {
                      frame False {
                        n4070 = local read "充电继电器"() -> (w5833:bool)
                        n4071 = Not(x=w5833) -> (.not. x?=w5834:bool)
                        n4072 = local write "充电继电器"(w5834) -> ()
                        n4073 = One Button Dialog(message="继电器处理超时" ("消息"), button name ("OK")="是" ("按钮名称（“确定”）")) -> ()  [unwired: 1 out]
                      }
                      frame True {
                      }
                    }
                  }
                }
              }
            }
          }
          event "风机继电器": Value Change {
            n4074 = event-data() -> ("NewVal"=w5837:bool)  [unwired: 6 out]
            n4075 = stacked-sequence {
              tunnel: w5837 -> [_ w5850 _]
              frame #0 {
                w5841 = FALSE ("继电器超时处理")
                n4076 = local write "继电器超时处理"(w5841) -> ()
                n4077 = local write "正级继电器 6"(w5841) -> ()
                n4078 = global write "EV05全局变量1.vi" "流控帧"(FALSE ("流控帧")) -> ()
                n4079 = local write "主从选择"(enum32{"主板", "从板"}."主板" ("主从选择")) -> ()
              }
              frame #1 {
                n4080 = case shown="真" w5850 {
                  selector: w5850 -> [w5864 w5884]
                  tunnel: [w5863 w5883] -> w5849
                  tunnel: [w5852 w5872] -> w5844
                  frame True {
                    w5860 = 256.0 ("y")
                    w5852 = u32 1 ("命令序号")
                    w5863 = u8 192 ("命令")
                    n4081 = local read "动作保持时间"() -> (w5861:dbl)
                    n4082 = Quotient & Remainder(x=w5861, y=w5860) -> (x-y*floor(x/y)=w5853:dbl, floor(x/y)=w5857:dbl)
                    n4083 = Quotient & Remainder(x=w5857, y=w5860) -> (x-y*floor(x/y)=w5854:dbl, floor(x/y)=w5858:dbl)
                    n4084 = Quotient & Remainder(x=w5858, y=w5860) -> (x-y*floor(x/y)=w5855:dbl, floor(x/y)=w5859:dbl)
                    n4085 = Boolean To (0,1)(Boolean=w5864) -> (0, 1=w5862:i16)
                    n4086 = local read "设备索引号"() -> (w5869:u16)
                    n4087 = local read "CAN卡类型"() -> (w5870:u32)
                    n4088 = Quotient & Remainder(x=w5859, y=w5860) -> (x-y*floor(x/y)=w5856:dbl)  [unwired: 1 out]
                    n4089 = local read "CAN端口"() -> (w5868:u16)
                    n4090 = Build Array(i16 6 ("元素"), w5862, w5856, w5855, w5854, w5853, 0.0 ("元素")) -> (w5866:dbl[])
                    n4091 = call "多帧发送机制(EV05).vi"("can卡类型"=w5870, "设备索引号"=w5869, "CAN端口"=w5868, "命令"=w5863, "板号"=u8 0, "命令序号"=w5852, "输入数据"=w5866) -> ()  [unwired: 2 in, 11 out]
                  }
                  frame False {
                    w5880 = 256.0 ("y")
                    w5872 = u32 1 ("命令序号")
                    w5883 = u8 192 ("命令")
                    n4092 = local read "动作保持时间"() -> (w5881:dbl)
                    n4093 = Quotient & Remainder(x=w5881, y=w5880) -> (x-y*floor(x/y)=w5873:dbl, floor(x/y)=w5877:dbl)
                    n4094 = Quotient & Remainder(x=w5877, y=w5880) -> (x-y*floor(x/y)=w5874:dbl, floor(x/y)=w5878:dbl)
                    n4095 = Quotient & Remainder(x=w5878, y=w5880) -> (x-y*floor(x/y)=w5875:dbl, floor(x/y)=w5879:dbl)
                    n4096 = Boolean To (0,1)(Boolean=w5884) -> (0, 1=w5882:i16)
                    n4097 = local read "设备索引号"() -> (w5889:u16)
                    n4098 = local read "CAN卡类型"() -> (w5890:u32)
                    n4099 = Quotient & Remainder(x=w5879, y=w5880) -> (x-y*floor(x/y)=w5876:dbl)  [unwired: 1 out]
                    n4100 = local read "CAN端口"() -> (w5888:u16)
                    n4101 = Build Array(i16 6 ("元素"), w5882, w5876, w5875, w5874, w5873, 0.0 ("元素")) -> (w5886:dbl[])
                    n4102 = call "多帧发送机制(EV05).vi"("can卡类型"=w5890, "设备索引号"=w5889, "CAN端口"=w5888, "命令"=w5883, "板号"=u8 0, "命令序号"=w5872, "输入数据"=w5886) -> ()  [unwired: 2 in, 11 out]
                  }
                }
                n4103 = local write "命令序号"(w5844) -> ()
                n4104 = local write "命令"(w5849) -> ()
                n4105 = local write "清BUFF"(FALSE ("清BUFF")) -> ()
                n4106 = local write "控制1"(TRUE ("控制1")) -> ()
                n4107 = global write "EV05全局变量1.vi" "流控帧 2"(TRUE ("流控帧 2")) -> ()
                n4108 = local write "写?"(FALSE ("写?")) -> ()
                n4109 = local write "消除"(TRUE ("消除")) -> ()
              }
              frame #2 {
                n4110 = flat-sequence {
                  tunnel: [w5892] -> w5891
                  tunnel: w5891 -> [w5899]
                  frame #0 {
                    n4111 = while {
                      tunnel: [w5893] -> w5892
                      i -> [w5897]
                      stop <- w5894 stop-if-true
                      n4112 = local read "继电器超时处理"() -> (w5893:bool)
                      n4113 = Greater Or Equal?(x=w5897, y=20) -> (x >= y?=w5895:bool)
                      n4114 = Wait Until Next ms Multiple(millisecond multiple=u32 100 ("毫秒倍数")) -> ()  [unwired: 1 out]
                      n4115 = Or(x=w5893, y=w5895) -> (x .or. y?=w5894:bool)
                    }
                  }
                  frame #1 {
                    n4116 = case shown="假" w5899 {
                      frame False {
                        n4117 = local read "风机继电器"() -> (w5900:bool)
                        n4118 = Not(x=w5900) -> (.not. x?=w5901:bool)
                        n4119 = local write "风机继电器"(w5901) -> ()
                        n4120 = One Button Dialog(message="继电器处理超时" ("消息"), button name ("OK")="是" ("按钮名称（“确定”）")) -> ()  [unwired: 1 out]
                      }
                      frame True {
                      }
                    }
                  }
                }
              }
            }
          }
          event "加热继电器(从)": Value Change {
            n4121 = event-data() -> ("NewVal"=w5904:bool)  [unwired: 6 out]
            n4122 = stacked-sequence {
              tunnel: w5904 -> [_ w5918 _]
              frame #0 {
                w5908 = FALSE ("继电器超时处理")
                n4123 = local write "正级继电器 7"(w5908) -> ()
                n4124 = local write "继电器超时处理"(w5908) -> ()
                n4125 = global write "EV05全局变量1.vi" "流控帧"(FALSE ("流控帧")) -> ()
                n4126 = local write "主从选择"(enum32{"主板", "从板"}."从板" ("主从选择")) -> ()
              }
              frame #1 {
                n4127 = case shown="真" w5918 {
                  selector: w5918 -> [w5933 w5953]
                  tunnel: [w5932 w5952] -> w5917
                  tunnel: [w5931 w5951] -> w5911
                  tunnel: [w5920 w5940] -> w5912
                  frame True {
                    w5928 = 256.0 ("y")
                    w5920 = u32 1 ("命令序号")
                    w5932 = u8 192 ("命令")
                    n4128 = local read "动作保持时间"() -> (w5929:dbl)
                    n4129 = Quotient & Remainder(x=w5929, y=w5928) -> (x-y*floor(x/y)=w5921:dbl, floor(x/y)=w5925:dbl)
                    n4130 = Quotient & Remainder(x=w5925, y=w5928) -> (x-y*floor(x/y)=w5922:dbl, floor(x/y)=w5926:dbl)
                    n4131 = Quotient & Remainder(x=w5926, y=w5928) -> (x-y*floor(x/y)=w5923:dbl, floor(x/y)=w5927:dbl)
                    n4132 = Quotient & Remainder(x=w5927, y=w5928) -> (x-y*floor(x/y)=w5924:dbl)  [unwired: 1 out]
                    n4133 = Boolean To (0,1)(Boolean=w5933) -> (0, 1=w5930:i16)
                    n4134 = local read "设备索引号"() -> (w5937:u16)
                    n4135 = local read "CAN卡类型"() -> (w5938:u32)
                    n4136 = local read "从板板号"() -> (w5931:u8)
                    n4137 = local read "CAN端口"() -> (w5936:u16)
                    n4138 = Build Array(i16 7 ("元素"), w5930, w5924, w5923, w5922, w5921, 0.0 ("元素")) -> (w5935:dbl[])
                    n4139 = call "多帧发送机制(EV05).vi"("can卡类型"=w5938, "设备索引号"=w5937, "CAN端口"=w5936, "命令"=w5932, "板号"=w5931, "命令序号"=w5920, "输入数据"=w5935) -> ()  [unwired: 2 in, 11 out]
                  }
                  frame False {
                    w5948 = 256.0 ("y")
                    w5940 = u32 1 ("命令序号")
                    w5952 = u8 192 ("命令")
                    n4140 = local read "动作保持时间"() -> (w5949:dbl)
                    n4141 = Quotient & Remainder(x=w5949, y=w5948) -> (x-y*floor(x/y)=w5941:dbl, floor(x/y)=w5945:dbl)
                    n4142 = Quotient & Remainder(x=w5945, y=w5948) -> (x-y*floor(x/y)=w5942:dbl, floor(x/y)=w5946:dbl)
                    n4143 = Quotient & Remainder(x=w5946, y=w5948) -> (x-y*floor(x/y)=w5943:dbl, floor(x/y)=w5947:dbl)
                    n4144 = Quotient & Remainder(x=w5947, y=w5948) -> (x-y*floor(x/y)=w5944:dbl)  [unwired: 1 out]
                    n4145 = Boolean To (0,1)(Boolean=w5953) -> (0, 1=w5950:i16)
                    n4146 = local read "设备索引号"() -> (w5957:u16)
                    n4147 = local read "CAN卡类型"() -> (w5958:u32)
                    n4148 = local read "从板板号"() -> (w5951:u8)
                    n4149 = local read "CAN端口"() -> (w5956:u16)
                    n4150 = Build Array(i16 7 ("元素"), w5950, w5944, w5943, w5942, w5941, 0.0 ("元素")) -> (w5955:dbl[])
                    n4151 = call "多帧发送机制(EV05).vi"("can卡类型"=w5958, "设备索引号"=w5957, "CAN端口"=w5956, "命令"=w5952, "板号"=w5951, "命令序号"=w5940, "输入数据"=w5955) -> ()  [unwired: 2 in, 11 out]
                  }
                }
                n4152 = local write "从板板号"(w5911) -> ()
                n4153 = local write "命令序号"(w5912) -> ()
                n4154 = local write "命令"(w5917) -> ()
                n4155 = local write "清BUFF"(FALSE ("清BUFF")) -> ()
                n4156 = local write "写?"(FALSE ("写?")) -> ()
                n4157 = local write "控制1"(TRUE ("控制1")) -> ()
                n4158 = global write "EV05全局变量1.vi" "流控帧 2"(TRUE ("流控帧 2")) -> ()
                n4159 = local write "消除"(TRUE ("消除")) -> ()
              }
              frame #2 {
                n4160 = flat-sequence {
                  tunnel: [w5960] -> w5959
                  tunnel: w5959 -> [w5967]
                  frame #0 {
                    n4161 = while {
                      tunnel: [w5961] -> w5960
                      i -> [w5965]
                      stop <- w5962 stop-if-true
                      n4162 = local read "继电器超时处理"() -> (w5961:bool)
                      n4163 = Greater Or Equal?(x=w5965, y=20) -> (x >= y?=w5963:bool)
                      n4164 = Wait Until Next ms Multiple(millisecond multiple=u32 100 ("毫秒倍数")) -> ()  [unwired: 1 out]
                      n4165 = Or(x=w5961, y=w5963) -> (x .or. y?=w5962:bool)
                    }
                  }
                  frame #1 {
                    n4166 = case shown="假" w5967 {
                      frame False {
                        n4167 = local read "加热继电器(从)"() -> (w5969:bool)
                        n4168 = Not(x=w5969) -> (.not. x?=w5968:bool)
                        n4169 = local write "加热继电器(从)"(w5968) -> ()
                        n4170 = One Button Dialog(message="继电器处理超时" ("消息"), button name ("OK")="是" ("按钮名称（“确定”）")) -> ()  [unwired: 1 out]
                      }
                      frame True {
                      }
                    }
                  }
                }
              }
            }
          }
          event "风机继电器(从)": Value Change {
            n4171 = event-data() -> ("NewVal"=w5972:bool)  [unwired: 6 out]
            n4172 = stacked-sequence {
              tunnel: w5972 -> [_ w5986 _]
              frame #0 {
                w5976 = FALSE ("继电器超时处理")
                n4173 = local write "继电器超时处理"(w5976) -> ()
                n4174 = local write "正级继电器 8"(w5976) -> ()
                n4175 = global write "EV05全局变量1.vi" "流控帧"(FALSE ("流控帧")) -> ()
                n4176 = local write "主从选择"(enum32{"主板", "从板"}."从板" ("主从选择")) -> ()
              }
              frame #1 {
                n4177 = case shown="假" w5986 {
                  selector: w5986 -> [w6001 w6021]
                  tunnel: [w6000 w6020] -> w5985
                  tunnel: [w5999 w6019] -> w5979
                  tunnel: [w5988 w6008] -> w5980
                  frame False {
                    w5996 = 256.0 ("y")
                    w5988 = u32 1 ("命令序号")
                    w6000 = u8 192 ("命令")
                    n4178 = local read "动作保持时间"() -> (w5997:dbl)
                    n4179 = Quotient & Remainder(x=w5997, y=w5996) -> (x-y*floor(x/y)=w5989:dbl, floor(x/y)=w5993:dbl)
                    n4180 = Quotient & Remainder(x=w5993, y=w5996) -> (x-y*floor(x/y)=w5990:dbl, floor(x/y)=w5994:dbl)
                    n4181 = Quotient & Remainder(x=w5994, y=w5996) -> (x-y*floor(x/y)=w5991:dbl, floor(x/y)=w5995:dbl)
                    n4182 = Quotient & Remainder(x=w5995, y=w5996) -> (x-y*floor(x/y)=w5992:dbl)  [unwired: 1 out]
                    n4183 = local read "设备索引号"() -> (w6005:u16)
                    n4184 = local read "CAN卡类型"() -> (w6006:u32)
                    n4185 = local read "从板板号"() -> (w5999:u8)
                    n4186 = Boolean To (0,1)(Boolean=w6001) -> (0, 1=w5998:i16)
                    n4187 = local read "CAN端口"() -> (w6004:u16)
                    n4188 = Build Array(i16 8 ("元素"), w5998, w5992, w5991, w5990, w5989, 0.0 ("元素")) -> (w6003:dbl[])
                    n4189 = call "多帧发送机制(EV05).vi"("can卡类型"=w6006, "设备索引号"=w6005, "CAN端口"=w6004, "命令"=w6000, "板号"=w5999, "命令序号"=w5988, "输入数据"=w6003) -> ()  [unwired: 2 in, 11 out]
                  }
                  frame True {
                    w6016 = 256.0 ("y")
                    w6008 = u32 1 ("命令序号")
                    w6020 = u8 192 ("命令")
                    n4190 = local read "动作保持时间"() -> (w6017:dbl)
                    n4191 = Quotient & Remainder(x=w6017, y=w6016) -> (x-y*floor(x/y)=w6009:dbl, floor(x/y)=w6013:dbl)
                    n4192 = Quotient & Remainder(x=w6013, y=w6016) -> (x-y*floor(x/y)=w6010:dbl, floor(x/y)=w6014:dbl)
                    n4193 = Quotient & Remainder(x=w6014, y=w6016) -> (x-y*floor(x/y)=w6011:dbl, floor(x/y)=w6015:dbl)
                    n4194 = Quotient & Remainder(x=w6015, y=w6016) -> (x-y*floor(x/y)=w6012:dbl)  [unwired: 1 out]
                    n4195 = local read "设备索引号"() -> (w6025:u16)
                    n4196 = local read "CAN卡类型"() -> (w6026:u32)
                    n4197 = local read "从板板号"() -> (w6019:u8)
                    n4198 = Boolean To (0,1)(Boolean=w6021) -> (0, 1=w6018:i16)
                    n4199 = local read "CAN端口"() -> (w6024:u16)
                    n4200 = Build Array(i16 8 ("元素"), w6018, w6012, w6011, w6010, w6009, 0.0 ("元素")) -> (w6023:dbl[])
                    n4201 = call "多帧发送机制(EV05).vi"("can卡类型"=w6026, "设备索引号"=w6025, "CAN端口"=w6024, "命令"=w6020, "板号"=w6019, "命令序号"=w6008, "输入数据"=w6023) -> ()  [unwired: 2 in, 11 out]
                  }
                }
                n4202 = local write "从板板号"(w5979) -> ()
                n4203 = local write "清BUFF"(FALSE ("清BUFF")) -> ()
                n4204 = local write "命令序号"(w5980) -> ()
                n4205 = local write "命令"(w5985) -> ()
                n4206 = local write "控制1"(TRUE ("控制1")) -> ()
                n4207 = local write "写?"(FALSE ("写?")) -> ()
                n4208 = local write "消除"(TRUE ("消除")) -> ()
                n4209 = global write "EV05全局变量1.vi" "流控帧 2"(TRUE ("流控帧 2")) -> ()
              }
              frame #2 {
                n4210 = flat-sequence {
                  tunnel: [w6028] -> w6027
                  tunnel: w6027 -> [w6035]
                  frame #0 {
                    n4211 = while {
                      tunnel: [w6029] -> w6028
                      i -> [w6033]
                      stop <- w6030 stop-if-true
                      n4212 = local read "继电器超时处理"() -> (w6029:bool)
                      n4213 = Greater Or Equal?(x=w6033, y=20) -> (x >= y?=w6031:bool)
                      n4214 = Wait Until Next ms Multiple(millisecond multiple=u32 100 ("毫秒倍数")) -> ()  [unwired: 1 out]
                      n4215 = Or(x=w6029, y=w6031) -> (x .or. y?=w6030:bool)
                    }
                  }
                  frame #1 {
                    n4216 = case shown="假" w6035 {
                      frame False {
                        n4217 = local read "风机继电器(从)"() -> (w6037:bool)
                        n4218 = Not(x=w6037) -> (.not. x?=w6036:bool)
                        n4219 = local write "风机继电器(从)"(w6036) -> ()
                        n4220 = One Button Dialog(message="继电器处理超时" ("消息"), button name ("OK")="是" ("按钮名称（“确定”）")) -> ()  [unwired: 1 out]
                      }
                      frame True {
                      }
                    }
                  }
                }
              }
            }
          }
          event "DO1": Value Change {
            n4221 = event-data() -> ("NewVal"=w6040:bool)  [unwired: 6 out]
            n4222 = stacked-sequence {
              tunnel: w6040 -> [_ w6053 _]
              frame #0 {
                w6043 = FALSE ("清BUFF")
                n4223 = local write "继电器超时处理"(FALSE ("继电器超时处理")) -> ()
                n4224 = local write "清BUFF"(w6043) -> ()
                n4225 = local write "正级继电器 9"(w6043) -> ()
                n4226 = local write "主从选择"(enum32{"主板", "从板"}."主板" ("主从选择")) -> ()
              }
              frame #1 {
                n4227 = case shown="真" w6053 {
                  selector: w6053 -> [w6068 w6088]
                  tunnel: [w6067 w6087] -> w6052
                  tunnel: [w6055 w6075] -> w6047
                  frame False {
                    w6063 = 256.0 ("y")
                    w6055 = u32 2 ("命令序号")
                    w6067 = u8 192 ("命令")
                    n4228 = local read "动作保持时间"() -> (w6064:dbl)
                    n4229 = Quotient & Remainder(x=w6064, y=w6063) -> (x-y*floor(x/y)=w6056:dbl, floor(x/y)=w6060:dbl)
                    n4230 = Quotient & Remainder(x=w6060, y=w6063) -> (x-y*floor(x/y)=w6057:dbl, floor(x/y)=w6061:dbl)
                    n4231 = Quotient & Remainder(x=w6061, y=w6063) -> (x-y*floor(x/y)=w6058:dbl, floor(x/y)=w6062:dbl)
                    n4232 = local read "设备索引号"() -> (w6072:u16)
                    n4233 = local read "CAN卡类型"() -> (w6073:u32)
                    n4234 = local read "CAN端口"() -> (w6071:u16)
                    n4235 = Boolean To (0,1)(Boolean=w6068) -> (0, 1=w6065:i16)
                    n4236 = Quotient & Remainder(x=w6062, y=w6063) -> (x-y*floor(x/y)=w6059:dbl)  [unwired: 1 out]
                    n4237 = Build Array(i16 1 ("元素"), w6065, w6059, w6058, w6057, w6056, 0.0 ("元素")) -> (w6069:dbl[])
                    n4238 = call "多帧发送机制(EV05).vi"("can卡类型"=w6073, "设备索引号"=w6072, "CAN端口"=w6071, "命令"=w6067, "板号"=u8 0, "命令序号"=w6055, "输入数据"=w6069) -> ()  [unwired: 2 in, 11 out]
                  }
                  frame True {
                    w6083 = 256.0 ("y")
                    w6075 = u32 2 ("命令序号")
                    w6087 = u8 192 ("命令")
                    n4239 = local read "动作保持时间"() -> (w6084:dbl)
                    n4240 = Quotient & Remainder(x=w6084, y=w6083) -> (x-y*floor(x/y)=w6076:dbl, floor(x/y)=w6080:dbl)
                    n4241 = Quotient & Remainder(x=w6080, y=w6083) -> (x-y*floor(x/y)=w6077:dbl, floor(x/y)=w6081:dbl)
                    n4242 = Quotient & Remainder(x=w6081, y=w6083) -> (x-y*floor(x/y)=w6078:dbl, floor(x/y)=w6082:dbl)
                    n4243 = local read "设备索引号"() -> (w6092:u16)
                    n4244 = local read "CAN卡类型"() -> (w6093:u32)
                    n4245 = local read "CAN端口"() -> (w6091:u16)
                    n4246 = Boolean To (0,1)(Boolean=w6088) -> (0, 1=w6085:i16)
                    n4247 = Quotient & Remainder(x=w6082, y=w6083) -> (x-y*floor(x/y)=w6079:dbl)  [unwired: 1 out]
                    n4248 = Build Array(i16 1 ("元素"), w6085, w6079, w6078, w6077, w6076, 0.0 ("元素")) -> (w6089:dbl[])
                    n4249 = call "多帧发送机制(EV05).vi"("can卡类型"=w6093, "设备索引号"=w6092, "CAN端口"=w6091, "命令"=w6087, "板号"=u8 0, "命令序号"=w6075, "输入数据"=w6089) -> ()  [unwired: 2 in, 11 out]
                  }
                }
